vi "List - Set Value to All.vi"(8 "Error In":errorcluster, 10 "Selected":bool, 11 "List In":string[](array[string])) -> (0 "Error Out":errorcluster, 3 "List Out":cluster{"Name":string, "Selected":bool}[](array[cluster]))   [LabVIEW 2020]
doc: "This VI use to set the value as False."
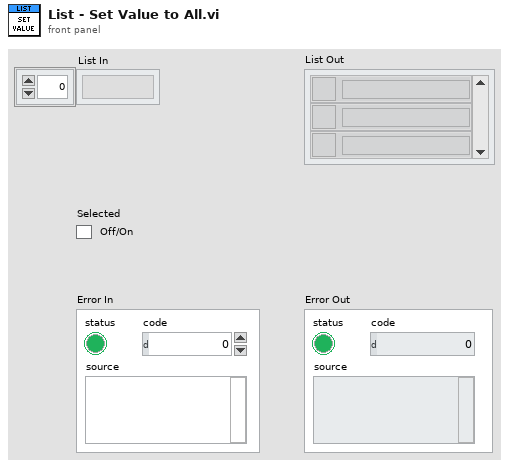
[diagram p1: front panel]
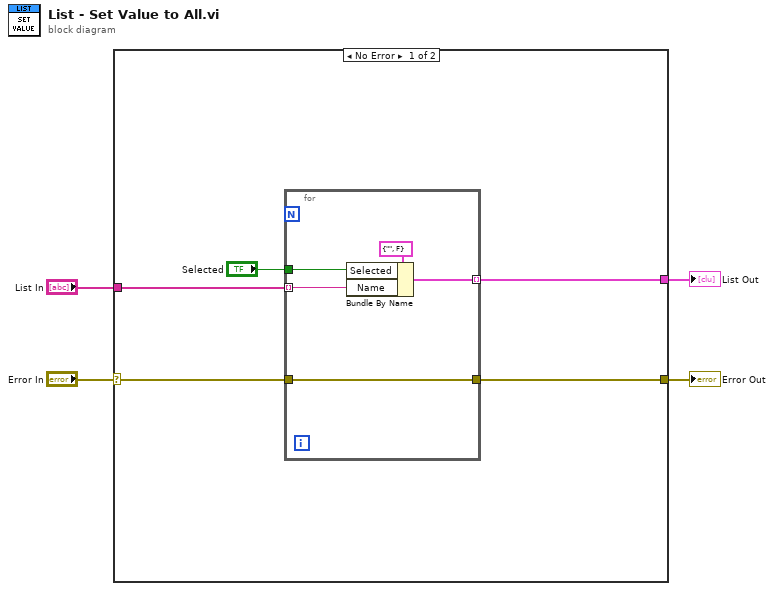
[diagram p0: block diagram]
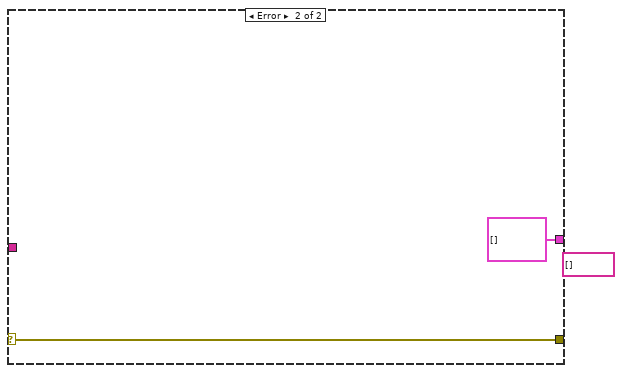
[diagram p2: hidden frame]
diagram:
  n1 = case shown="No Error" "Error In" {
    selector: "Error In" -> [w9 w16]
    tunnel: [w8 w16] -> w3
    tunnel: "List In" -> [w7 _]
    tunnel: [w6 cluster{"Name":string, "Selected":bool}[] []] -> w1
    frame No Error {
      n2 = for {
        tunnel: w7 -> [w13] mode=indexing
        tunnel: [w14] -> w8
        tunnel: w9 -> [w14]
        tunnel: [w11] -> w6 mode=indexing
        tunnel: "Selected" -> [w10]
        n3 = Bundle By Name(cluster=cluster{"Name":string, "Selected":bool} {"Name"="", "Selected"=FALSE} ("File List"), "Selected"=w10, "Name"=w13) -> (w11:cluster{"Name":string, "Selected":bool})
      }
    }
    frame Error {
      (unwired) string[] []
      (unwired) string[] []
    }
  }
  "Error Out" <- w3
  "List Out" <- w1
